vi "rngtest.vi"() -> ()   [LabVIEW 2025]
panel:
  out "round":u32
  in  "size":i32
  in  "layers":i32
  out "real count":i32
  in  "mine count":i32
  out "good":bool
  # "checking rng mine count"
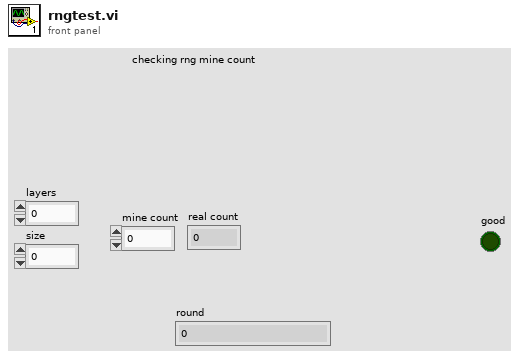
[diagram p1: front panel]
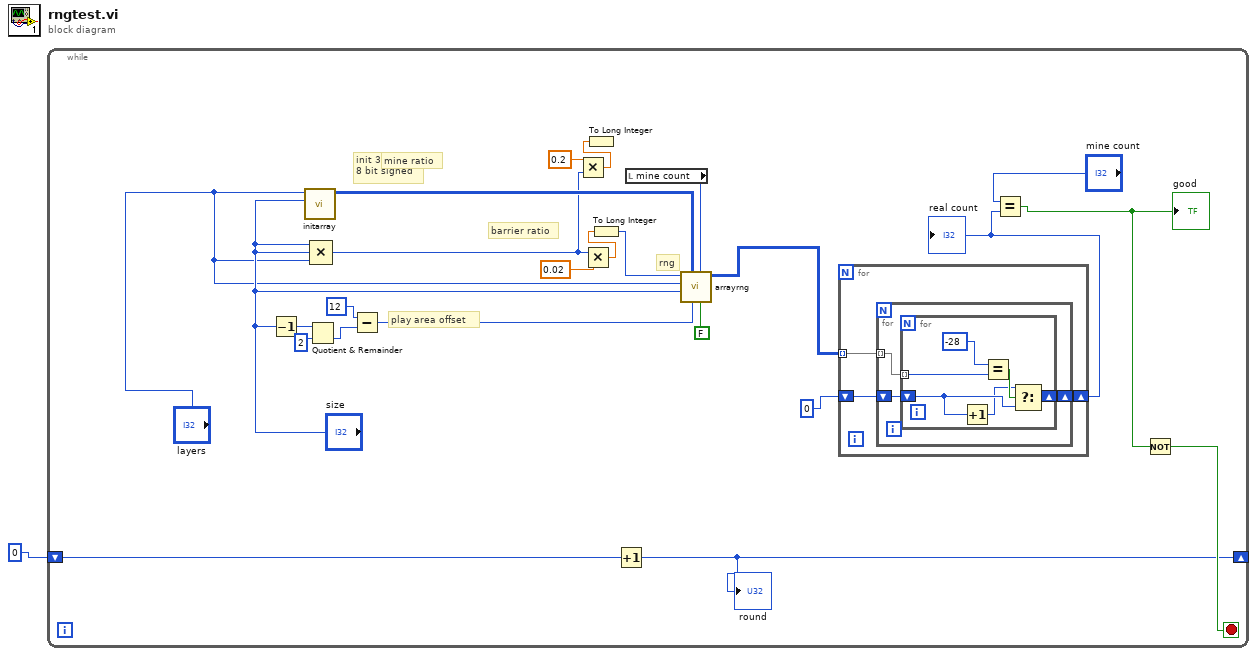
[diagram p0: block diagram]
diagram:
  n1 = while {
    shift-right: [w2] -> _
    shift-left: u32 0 -> [w3]
    stop <- w4 stop-if-true
    # "play area offset"
    # "rng"
    # "barrier ratio"
    # "mine ratio"
    # "init 3d array\n8 bit signed"
    n2 = Decrement(x="size") -> (x-1=w11:i32)
    n3 = call "initarray.vi"("size"="size", "layers"="layers") -> ("Array"=w19:i8[][][])  [unwired: 9 in]
    n4 = Quotient & Remainder(x=w11, y=2) -> (floor(x/y)=w10:i32)  [unwired: 1 out]
    n5 = Compound Arithmetic op=MULTIPLY("size", "size", "layers") -> (w13:i32)
    n6 = Subtract(x=12, y=w10) -> (x-y=w9:i32)
    n7 = Multiply(x=0.2 ("y"), y=w13) -> (x*y=w17:dbl)
    n8 = Multiply(x=w13, y=0.02) -> (x*y=w15:dbl)
    n9 = To Long Integer(number=w17) -> ()  [unwired: 1 out]
    n10 = To Long Integer(number=w15) -> (32bit integer=w16:i32)
    n11 = Increment(x=w3) -> (x+1=w2:u32)
    "round" <- w2
    n12 = local read "mine count"() -> (w7:i32)
    n13 = call "arrayrng.vi"("barrier?"=FALSE ("barrier"), "mine count"=w7, "sizeoffset"=w9, "empty array"=w19, "size"="size", "layers"="layers", "barrier count"=w16) -> ("Array out"=w20:i8[][][])  [unwired: 4 in]
    n14 = for {
      tunnel: w20 -> [w28] mode=indexing
      shift-right: [w26] -> w24
      shift-left: 0 -> [w27]
      n15 = for {
        tunnel: w28 -> [w29] mode=indexing
        shift-right: [w31] -> w26
        shift-left: w27 -> [w30]
        n16 = for {
          shift-right: [w36] -> w31
          shift-left: w30 -> [w35]
          tunnel: w29 -> [w32] mode=indexing
          n17 = Increment(x=w35) -> (x+1=w34:i32)
          n18 = Equal?(x=i8 -28 ("element"), y=w32) -> (x = y?=w37:bool)
          n19 = Select(t=w34, s=w37, f=w35) -> (s? t:f=w36:i32)
        }
      }
    }
    "real count" <- w24
    n20 = Equal?(x="mine count", y=w24) -> (x = y?=w5:bool)
    "good" <- w5
    n21 = Not(x=w5) -> (.not. x?=w4:bool)
  }
